vi "acc_gyro to waveform.vi"(11 "acc gyro data":T1) -> (2 "accel plot":waveform(dbl)[](array[waveform]), 3 "gyro plot":waveform(dbl)[](array[waveform]))   [LabVIEW 2012]
uses:
  acc_gyro_data.ctl
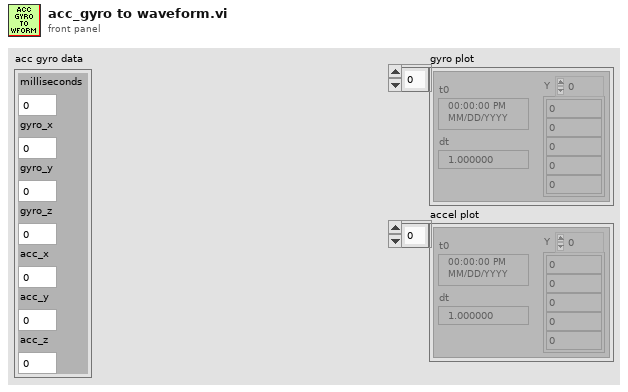
[diagram p1: front panel]
types:
  T1 = typedef "acc_gyro_data.ctl" = cluster{"milliseconds":u64, "gyro_x":dbl, "gyro_y":dbl, "gyro_z":dbl, "acc_x":dbl, "acc_y":dbl, "acc_z":dbl}
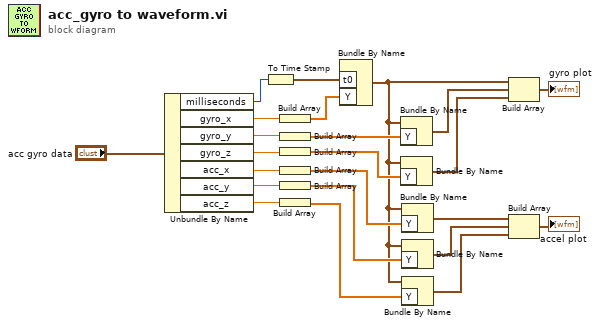
[diagram p0: block diagram]
diagram:
  n1 = Unbundle By Name("acc gyro data") -> ("milliseconds"=w22:u64, "gyro_x"=w20:dbl, "gyro_y"=w18:dbl, "gyro_z"=w17:dbl, "acc_x"=w16:dbl, "acc_y"=w15:dbl, "acc_z"=w14:dbl)
  n2 = To Time Stamp(1:w22) -> (0:w21:timestamp)
  n3 = Build Array(w20) -> (w19:dbl[])
  n4 = Build Array(w18) -> (w13:dbl[])
  n5 = Build Array(w17) -> (w12:dbl[])
  n6 = Build Array(w16) -> (w11:dbl[])
  n7 = Build Array(w15) -> (w10:dbl[])
  n8 = Build Array(w14) -> (w9:dbl[])
  n9 = Bundle By Name("t0"=w21, "Y"=w19) -> (w8:waveform(dbl))  [unwired: 1 in]
  n10 = Bundle By Name(cluster=w8, "Y"=w13) -> (w7:waveform(dbl))
  n11 = Bundle By Name(cluster=w8, "Y"=w12) -> (w6:waveform(dbl))
  n12 = Bundle By Name(cluster=w8, "Y"=w11) -> (w5:waveform(dbl))
  n13 = Bundle By Name(cluster=w8, "Y"=w10) -> (w4:waveform(dbl))
  n14 = Bundle By Name(cluster=w8, "Y"=w9) -> (w3:waveform(dbl))
  n15 = Build Array(w8, w7, w6) -> (→"gyro plot":waveform(dbl)[])
  n16 = Build Array(w5, w4, w3) -> (→"accel plot":waveform(dbl)[])
